vi "MB Slave Write Discrete Inputs (poly).vi"(1 "Starting Address":u16, 2 "Discrete Inputs":bool[](array[boolean]), 5 "error in":errorcluster) -> (19 "error out":errorcluster)   [LabVIEW 2020]
doc: "Writes multiple discrete inputs to the slave memory tables."
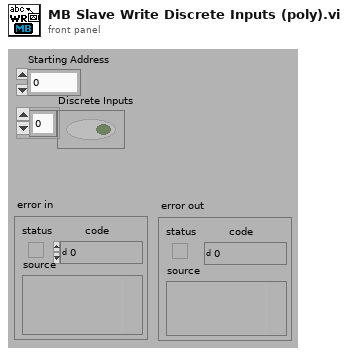
[diagram p1: front panel]
types:
  T1 = enum16{"Discrete Inputs", "Coils", "Input Registers", "Holding Registers"}
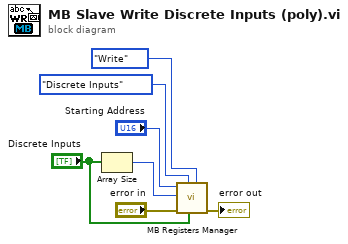
[diagram p0: block diagram]
diagram:
  n1 = Array Size(array="Discrete Inputs") -> (size(s)=w1:i32)
  n2 = call "MB Registers Manager.vi"("Function"=enum16{"Init", "Read", "Write", "Read All"}."Write", "Bits In"="Discrete Inputs", "Table"=T1."Discrete Inputs", "error in (no error)"="error in", "Length"=w1, "Start Address"="Starting Address") -> ("error out"=→"error out":errorcluster)  [unwired: 1 in, 4 out]
